vi "Quit GNU Octave.vi"(8 "error in":errorcluster, 11 "pipe in":T1) -> (0 "error out":errorcluster, 2 "exit code":i32)   [LabVIEW 2013, in "GOLPI library.lvlib"]
uses:
  GOLPI library.lvlib
  LV Process.lvlibp/Pipe Handle.ctl
  LV Process.lvlibp
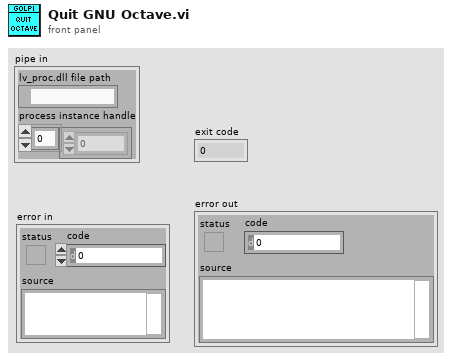
[diagram p1: front panel]
types:
  T1 = typedef "LV Process.lvlibp/Pipe Handle.ctl" = cluster{"lv_proc.dll file path":path, "process instance handle":u32[]}
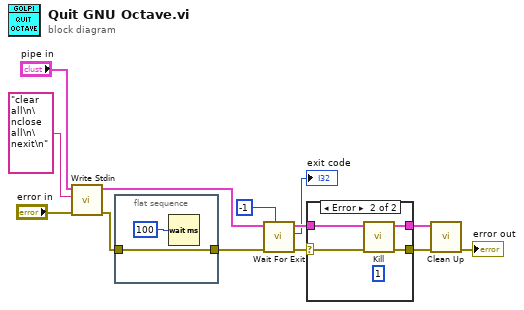
[diagram p0: block diagram]
diagram:
  n1 = call "Write Stdin.vi"("error in"="error in", "write buffer"="clear all\n\nclose all\n\nexit\n", "pipe in"="pipe in") -> ("error out"=w2:errorcluster, "pipe out"=w1:T1)  [unwired: 6 in, 1 out]
  n2 = flat-sequence {
    tunnel: [w14] -> w3
    tunnel: w2 -> [w14]
    frame #0 {
      n3 = Wait (ms)(milliseconds to wait=u32 100) -> ()  [unwired: 1 out]
    }
  }
  n4 = call "Wait For Exit.vi"("timeout [ms]"=-1, "error in"=w3, "pipe in"=w1) -> ("error out"=w11:errorcluster, "exit code"=→"exit code":i32, "pipe out"=w10:T1)  [unwired: 6 in]
  n5 = case shown="Error" w11 {
    selector: w11 -> [w16 w20]
    tunnel: w10 -> [w17 w19]
    tunnel: [w16 w21] -> w12
    tunnel: [w17 w18] -> w8
    frame No Error {
    }
    frame Error {
      (unwired) 1 ("timeout [ms]")
      n6 = call "Kill.vi"("error in"=w20, "pipe in"=w19) -> ("error out"=w21:errorcluster, "pipe out"=w18:T1)  [unwired: 8 in]
    }
  }
  n7 = call "Clean Up.vi"("error in"=w12, "pipe in"=w8) -> ("error out"=→"error out":errorcluster)  [unwired: 9 in]
